vi "Set Light On.vi"(8 "error in (no error)":errorcluster, 9 "On":bool, 10 "Light Selection":T1, 11 "LightsPanel in":refnum<class "LightsPanel.lvclass">) -> (0 "error out":errorcluster, 3 "LightsPanel out":refnum<class "LightsPanel.lvclass">)   [LabVIEW 2022 SP3, in "TouchControl.lvlib" / "LightsPanel.lvclass"]
uses:
  LightsPanel.lvclass
  Light Selection.ctl
  TouchControl.lvlib
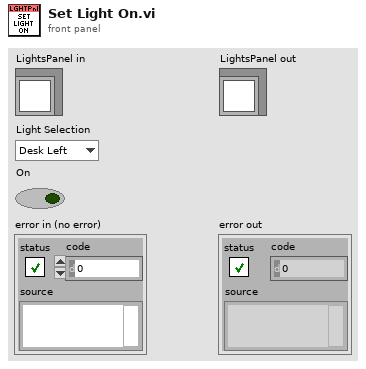
[diagram p1: front panel]
types:
  T1 = typedef "TouchControl.lvlib/Light Selection.ctl" = enum16{"Desk Left", "Desk Right", "Printer"}
  T2 = typedef "TouchControl.lvlib/Light Config.ctl" = cluster{"Desk Left":string, "Desk Right":string, "Printer":string}
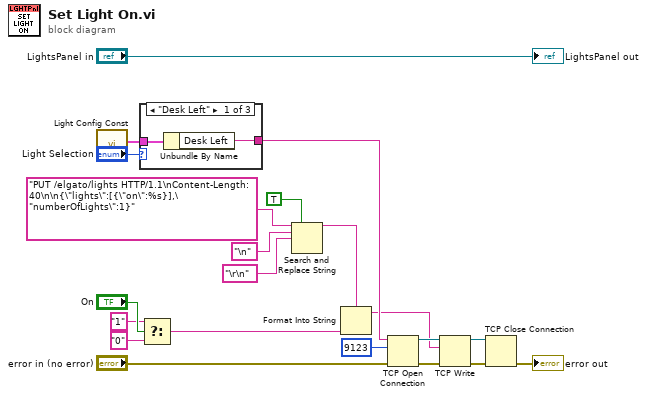
[diagram p0: block diagram]
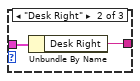
[diagram p2: hidden frame]
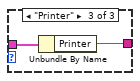
[diagram p3: hidden frame]
diagram:
  n1 = call "Light Config Const.vi"() -> ("Light Config"=w19:T2)  [unwired: 11 in]
  n2 = case shown="\"Desk Left\"" "Light Selection" {
    tunnel: w19 -> [w23 w25 w27]
    tunnel: [w22 w24 w26] -> w13
    frame "Desk Left" {
      n3 = Unbundle By Name(w23) -> ("Desk Left"=w22:string)
    }
    frame "Desk Right" {
      n4 = Unbundle By Name(w25) -> ("Desk Right"=w24:string)
    }
    frame "Printer" {
      n5 = Unbundle By Name(w27) -> ("Printer"=w26:string)
    }
  }
  n6 = Select(t="1", s="On", f="0") -> (s? t:f=w15:string)
  n7 = Search and Replace String(replace all?=TRUE ("replace all? (F)"), input string="PUT /elgato/lights HTTP/1.1\nContent-Length: 40\n\n{\"lights\":[{\"on\":%s}],\"numberOfLights\":1}", search string="\n", replace string="\r\n" ("search string")) -> (result string=w4:string)  [unwired: 4 in, 3 out]
  n8 = Format Into String(format string=w4, w15) -> (resulting string=w3:string)  [unwired: 2 in, 1 out]
  n9 = TCP Open Connection(address=w13, remote port or service name=u16 9123, error in (no error)="error in (no error)") -> (connection ID=w10:refnum<k5>, error out=w11:errorcluster)  [unwired: 2 in]
  n10 = TCP Write(connection ID=w10, data in=w3, error in (no error)=w11) -> (connection ID out=w2:refnum<k5>, error out=w1:errorcluster)  [unwired: 1 in, 1 out]
  n11 = TCP Close Connection(connection ID=w2, error in (no error)=w1) -> (error out=→"error out":errorcluster)  [unwired: 1 in, 1 out]
  "LightsPanel out" <- "LightsPanel in"
